vi "test Error Propagation.vi"(8 "error in":errorcluster, 11 "TestCase in":refnum<class "Scripting.lvclass">) -> (0 "error out":errorcluster, 3 "TestCase out":refnum<class "Scripting.lvclass">)   [LabVIEW 2023, in "Scripting.lvclass"]
uses:
  Scripting.lvclass
  Scripting.lvclass/Scripting.ctl
  <vilib>/addons/_JKI Toolkits/VI Tester/TestCase.llb/TestCase.lvclass
  Scripting/Ballard MIL-STD-1553 Scripting.lvlib
  <vilib>/NI VeriStand/Custom Device API/Custom Device Item Ref.ctl
  <vilib>/NI VeriStand/Custom Device API/Custom Device API.lvlib
  Shared/Address.ctl
  Shared/Terminal Endpoint.ctl
  Shared/Parameter Definition.ctl
  Shared/Message Type.ctl
  Shared/Message Definition.ctl
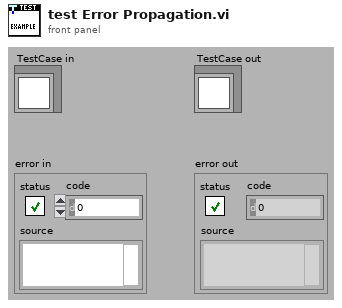
[diagram p1: front panel]
types:
  T1 = typedef "Custom Device API.lvlib/Custom Device Item Ref.ctl" = u64
  T2 = typedef "Message Definition.ctl" = cluster{"name":string, "message type":T3, "endpoint Tx":T4, "endpoint Rx":T4, "create timestamp channel":bool, "mode code":u16, "number of words":u16, "parameters":cluster{"name":string, "default value":dbl, "unit":string, "parameter definition":T6}[]}
  T3 = typedef "Message Type.ctl" = string
  T4 = typedef "Terminal Endpoint.ctl" = cluster{"terminal address":T5, "subaddress":T5}
  T5 = typedef "Address.ctl" = u16
  T6 = typedef "Parameter Definition.ctl" = cluster{"start index":i32, "size (bits)":i32, "encoding":enum16{"BNR", "BCD", "Discrete"}, "signed":bool, "multiplier":dbl, "offset":dbl}
  T7 = cluster{"Rx remote terminal":T4, "Rx remote terminal":T4}
  T8 = typedef "Device Parameters.ctl" = cluster{"initialization method":T9, "card number":i32, "PXI slot number":i32, "core number":i32}
  T9 = typedef "Initialization Method.ctl" = enum16{"PXI Slot Number", "Card Number"}
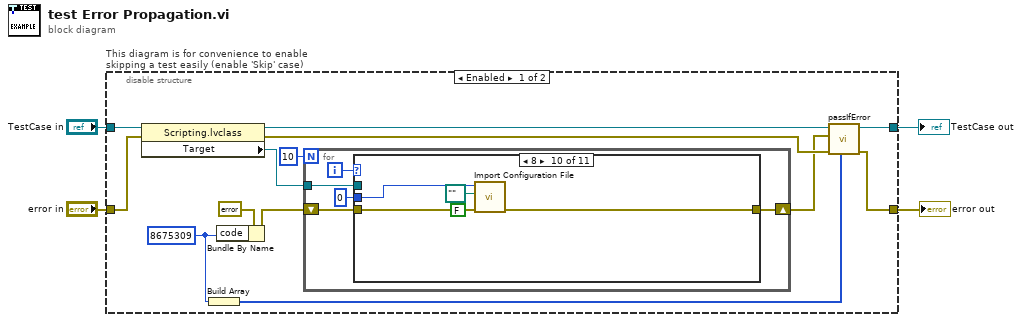
[diagram p0: block diagram]
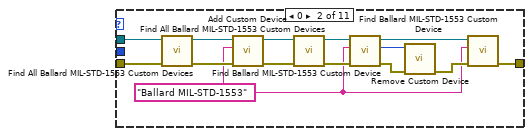
[diagram p3: hidden frame]
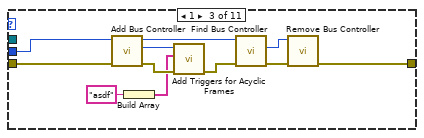
[diagram p4: hidden frame]
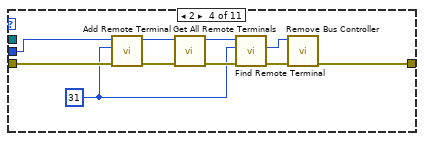
[diagram p5: hidden frame]
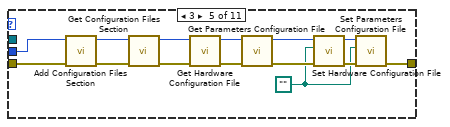
[diagram p6: hidden frame]
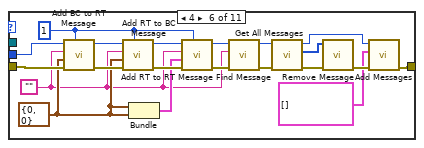
[diagram p7: hidden frame]
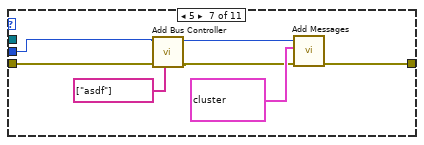
[diagram p8: hidden frame]
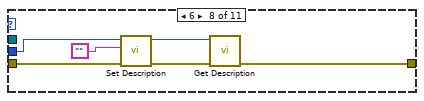
[diagram p9: hidden frame]
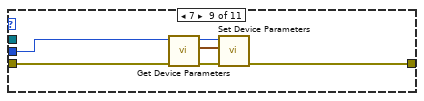
[diagram p10: hidden frame]
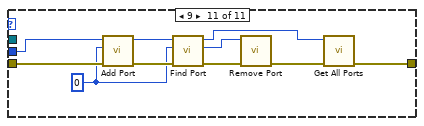
[diagram p11: hidden frame]
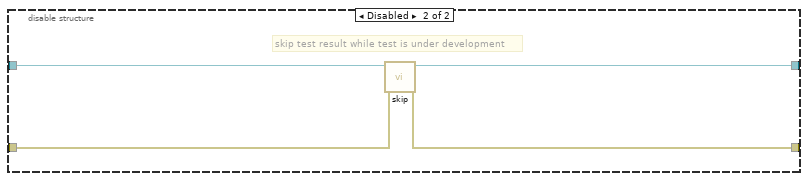
[diagram p12: hidden frame]
diagram:
  n1 = disable-structure "This diagram is for convenience to enable skipping a test easily (enable 'Skip' case)" shown="Enabled" {
    disable-tunnel: "TestCase in" -> [w15 w130]
    disable-tunnel: [w17 w128] -> w1
    disable-tunnel: [w16 w129] -> w3
    disable-tunnel: "error in" -> [w12 w127]
    frame Enabled {
      w8 = 8675309 ("code")
      n2 = property class="Scripting.lvclass"(reference=w15, error in=w12) -> (reference out=w14:refnum<class "Scripting.lvclass">, error out=w11:errorcluster, "Target"=w13:refnum<k24>)
      n3 = Build Array(w8) -> (w7:i32[])
      n4 = Bundle By Name(cluster=errorcluster {"status"=TRUE, "code"=-9999, "source"=""} ("error in"), "code"=w8) -> (w9:errorcluster)
      n5 = for {
        N: 10 -> [_]
        tunnel: w13 -> [w22]
        shift-right: [w20] -> w6
        shift-left: w9 -> [w21]
        i -> [w19]
        n6 = case shown="8" w19 {
          tunnel: w22 -> [_ w26 _ _ _ _ _ _ _ _ _]
          tunnel: w21 -> [w23 w25 w48 w58 w72 w83 w97 w105 w107 w115 w121]
          tunnel: [w23 w24 w46 w54 w62 w75 w99 w101 w106 w114 w120] -> w20
          tunnel: T1 0 ("Ballard MIL-STD 1553 custom device in") -> [_ _ w38 w49 w59 w77 w94 w104 w108 w116 w119]
          frame Default {
          }
          frame 0 {
            w28 = "Ballard MIL-STD-1553" ("name")
            n7 = call "Find All Ballard MIL-STD-1553 Custom Devices.vi"("error in"=w25, "target in"=w26) -> ("error out"=w37:errorcluster, "target out"=w36:refnum<k24>)  [unwired: 7 in, 1 out]
            n8 = call "Add Custom Device.vi"("error in"=w37, "name"=w28, "target in"=w36) -> ("error out"=w35:errorcluster, "target out"=w34:refnum<k24>)  [unwired: 6 in, 1 out]
            n9 = call "Find All Ballard MIL-STD-1553 Custom Devices.vi"("error in"=w35, "target in"=w34) -> ("error out"=w33:errorcluster, "target out"=w32:refnum<k24>)  [unwired: 7 in, 1 out]
            n10 = call "Find Ballard MIL-STD-1553 Custom Device.vi"("error in"=w33, "name"=w28, "target in"=w32) -> ("error out"=w31:errorcluster, "Ballard MIL-STD 1553 custom device"=w30:T1, "target out"=w27:refnum<k24>)  [unwired: 5 in, 1 out]
            n11 = call "Remove Custom Device.vi"("error in"=w31, "Ballard MIL-STD 1553 custom device"=w30) -> ("error out"=w29:errorcluster)  [unwired: 9 in]
            n12 = call "Find Ballard MIL-STD-1553 Custom Device.vi"("error in"=w29, "name"=w28, "target in"=w27) -> ("error out"=w24:errorcluster)  [unwired: 5 in, 3 out]
          }
          frame 1 {
            n13 = call "Add Bus Controller.vi"("error in"=w48, "port in"=w38) -> ("error out"=w42:errorcluster, "bus controller"=w43:T1, "port out"=w45:T1)  [unwired: 7 in]
            n14 = Build Array("asdf" ("acyclic buffer name")) -> (w39:string[])
            n15 = call "Add Triggers for Acyclic Frames.vi"("error in"=w42, "acyclic frame names"=w39, "bus controller in"=w43) -> ("error out"=w41:errorcluster)  [unwired: 7 in, 1 out]
            n16 = call "Find Bus Controller.vi"("error in"=w41, "port in"=w45) -> ("error out"=w47:errorcluster, "bus controller"=w44:T1)  [unwired: 6 in, 2 out]
            n17 = call "Remove Bus Controller.vi"("error in"=w47, "bus controller"=w44) -> ("error out"=w46:errorcluster)  [unwired: 9 in]
          }
          frame 2 {
            w50 = T5 31 ("terminal address")
            n18 = call "Add Remote Terminal.vi"("error in"=w58, "terminal address"=w50, "port in"=w49) -> ("error out"=w57:errorcluster, "port out"=w52:T1)  [unwired: 6 in, 1 out]
            n19 = call "Get All Remote Terminals.vi"("error in"=w57, "port in"=w52) -> ("error out"=w56:errorcluster, "port out"=w51:T1)  [unwired: 7 in, 1 out]
            n20 = call "Find Remote Terminal.vi"("error in"=w56, "terminal address"=w50, "port in"=w51) -> ("error out"=w55:errorcluster, "remote terminal"=w53:T1)  [unwired: 5 in, 2 out]
            n21 = call "Remove Bus Controller.vi"("error in"=w55, "bus controller"=w53) -> ("error out"=w54:errorcluster)  [unwired: 9 in]
          }
          frame 3 {
            w61 = path ""
            n22 = call "Add Configuration Files Section.vi"("error in"=w72, "custom device in"=w59) -> ("error out"=w71:errorcluster, "custom device out"=w67:T1)  [unwired: 7 in, 1 out]
            n23 = call "Get Configuration Files Section.vi"("error in"=w71, "custom device in"=w67) -> ("error out"=w70:errorcluster, "custom device out"=w66:T1)  [unwired: 6 in, 2 out]
            n24 = call "Get Hardware Configuration File.vi"("error in"=w70, "Ballard MIL-STD 1553 custom device in"=w66) -> ("error out"=w69:errorcluster, "Ballard MIL_STD 1553 custom device out"=w68:T1)  [unwired: 6 in, 2 out]
            n25 = call "Get Parameters Configuration File.vi"("error in"=w69, "Ballard MIL-STD 1553 custom device in"=w68) -> ("error out"=w63:errorcluster, "Ballard MIL-STD 1553 custom device out"=w60:T1)  [unwired: 6 in, 2 out]
            n26 = call "Set Hardware Configuration File.vi"("error in"=w63, "hardware configuration file path"=w61, "Ballard MIL-STD 1553 custom device in"=w60) -> ("error out"=w65:errorcluster, "Ballard MIL-STD 1553 custom device out"=w64:T1)  [unwired: 7 in]
            n27 = call "Set Parameters Configuration File.vi"("error in"=w65, "parameters configuration file path"=w61, "Ballard MIL-STD 1553 custom device in"=w64) -> ("error out"=w62:errorcluster)  [unwired: 7 in, 1 out]
          }
          frame 4 {
            w80 = T4 {"terminal address"=0, "subaddress"=0} ("Rx remote terminal")
            w78 = "" ("name")
            w81 = u16 1 ("number of words")
            n28 = call "Add BC to RT Message.vi"("number of words"=w81, "error in"=w83, "Rx remote terminal"=w80, "name"=w78, "port in"=w77) -> ("error out"=w91:errorcluster, "port out"=w92:T1)  [unwired: 3 in, 2 out]
            n29 = call "Add RT to BC Message.vi"("number of words"=w81, "error in"=w91, "Tx remote terminal"=w80, "name"=w78, "port in"=w92) -> ("error out"=w89:errorcluster, "port out"=w90:T1)  [unwired: 3 in, 2 out]
            n30 = Bundle("Rx remote terminal"=w80, "Rx remote terminal"=w80) -> (w79:T7)  [unwired: 1 in]
            n31 = call "Add RT to RT Message.vi"("number of words"=w81, "error in"=w89, "remote terminals"=w79, "name"=w78, "port in"=w90) -> ("error out"=w87:errorcluster, "port out"=w88:T1)  [unwired: 4 in, 1 out]
            n32 = call "Find Message.vi"("error in"=w87, "message name"=w78, "port in"=w88) -> ("error out"=w85:errorcluster, "port out"=w86:T1)  [unwired: 5 in, 2 out]
            n33 = call "Get All Messages.vi"("error in"=w85, "port in"=w86) -> ("error out"=w84:errorcluster, "messages"=w82:T1[], "port out"=w74:T1)  [unwired: 7 in]
            n34 = call "Remove Message.vi"("error in"=w84, "message refs"=w82) -> ("error out"=w76:errorcluster)  [unwired: 9 in]
            n35 = call "Add Messages.vi"("error in"=w76, "messages"=T2[] [], "port in"=w74) -> ("error out"=w75:errorcluster)  [unwired: 7 in, 1 out]
          }
          frame 5 {
            n36 = call "Add Bus Controller.vi"("acyclic frame names"=string[] ["asdf"], "error in"=w97, "port in"=w94) -> ("error out"=w96:errorcluster, "port out"=w95:T1)  [unwired: 6 in, 1 out]
            n37 = call "Add Messages.vi"("error in"=w96, "messages"=T2[] [{"name"="", "message type"="BC to RT", "endpoint Tx"={"terminal address"=0, "subaddress"=0}, "endpoint Rx"={"terminal address"=0, "subaddress"=0}, "create timestamp channel"=FALSE, "mode code"=0, "number of words"=0, "parameters"=[{"name"="p0", "default value"=1.0, "unit"="", "parameter definition"={"start index"=0, "size (bits)"=16, "encoding"=enum."BNR", "signed"=TRUE, "multiplier"=1.0, "offset"=0.0}}]}], "port in"=w95) -> ("error out"=w99:errorcluster)  [unwired: 7 in, 1 out]
          }
          frame 6 {
            n38 = call "Set Description.vi"("error in"=w105, "description"="", "Ballard MIL-STD 1553 custom device in"=w104) -> ("error out"=w103:errorcluster, "Ballard MIL-STD 1553 custom device out"=w102:T1)  [unwired: 7 in]
            n39 = call "Get Description.vi"("error in"=w103, "Ballard MIL-STD 1553 custom device in"=w102) -> ("error out"=w101:errorcluster)  [unwired: 7 in, 2 out]
          }
          frame 7 {
            n40 = call "Get Device Parameters.vi"("error in"=w107, "Ballard MIL-STD 1553 custom device in"=w108) -> ("error out"=w110:errorcluster, "device parameters"=w109:T8, "Ballard MIL-STD 1553 custom device out"=w111:T1)  [unwired: 7 in]
            n41 = call "Set Device Parameters.vi"("error in"=w110, "device parameters"=w109, "Ballard MIL-STD 1553 custom device in"=w111) -> ("error out"=w106:errorcluster)  [unwired: 7 in, 1 out]
          }
          frame 8 {
            n42 = call "Import Configuration File.vi"("error in"=w115, "create Tx/Rx folders for subaddresses?"=FALSE, "parameters configuration file path"=path "", "Ballard MIL-STD 1553 custom device in"=w116) -> ("error out"=w114:errorcluster)  [unwired: 6 in, 1 out]
          }
          frame 9 {
            w118 = u16 0 ("port number")
            n43 = call "Add Port.vi"("error in"=w121, "port number"=w118, "Ballard MIL-STD 1553 custom device in"=w119) -> ("error out"=w125:errorcluster, "Ballard MIL-STD 1553 custom device out"=w126:T1)  [unwired: 6 in, 1 out]
            n44 = call "Find Port.vi"("error in"=w125, "port number"=w118, "Ballard MIL-STD 1553 custom device in"=w126) -> ("error out"=w124:errorcluster, "port"=w122:T1, "Ballard MIL-STD 1553 custom device out"=w117:T1)  [unwired: 5 in, 1 out]
            n45 = call "Remove Port.vi"("error in"=w124, "port"=w122) -> ("error out"=w123:errorcluster)  [unwired: 9 in]
            n46 = call "Get All Ports.vi"("error in"=w123, "Ballard MIL-STD 1553 custom device in"=w117) -> ("error out"=w120:errorcluster)  [unwired: 7 in, 2 out]
          }
        }
      }
      n47 = call-dynamic "passIfError.vi"("passing error codes (default = any error code)"=w7, "error in (no error)"=w11, "error"=w6, "TestCase in"=w14) -> ("error out"=w16:errorcluster, "TestCase out"=w17:refnum<class "Scripting.lvclass">)  [unwired: 6 in]
    }
    frame Disabled {
      # "skip test result while test is under development"
      n48 = call <vilib>:"skip.vi"("error in (no error)"=w127, "TestCase in"=w130) -> ("error out"=w129:errorcluster, "TestCase out"=w128:refnum<class "Scripting.lvclass">)  [unwired: 8 in]
    }
  }
  "error out" <- w3
  "TestCase out" <- w1
